vi "read from connection.vi"(8 "error in":errorcluster, 9 "timeout ms (-1)":i32=-1, 11 "connection in":refnum<class "connection maintainer.lvclass">) -> (0 "error out":errorcluster, 1 "valid?":bool, 2 "data message":refnum<class "communicator message.lvclass">, 3 "connection out":refnum<class "connection maintainer.lvclass">)   [LabVIEW 2015, in "connection maintainer.lvclass"]
uses:
  connection maintainer.lvclass
  message/communicator message.lvclass
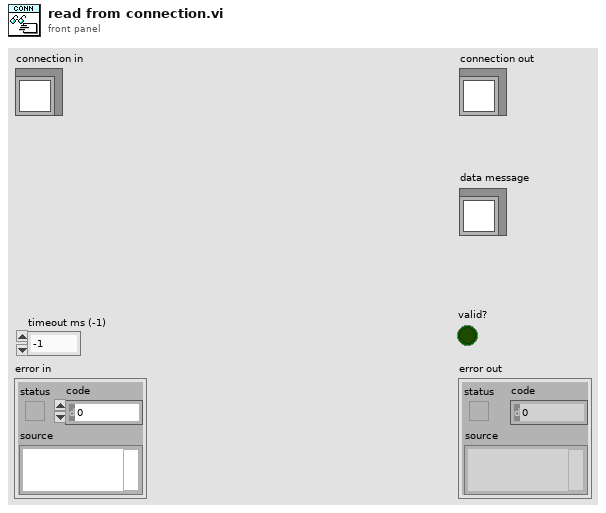
[diagram p1: front panel]
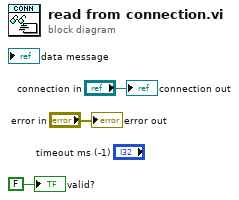
[diagram p0: block diagram]
diagram:
  "error out" <- "error in"
  "connection out" <- "connection in"
  "valid?" <- FALSE ("valid?")
